vi "form FP title.vi"(2 "object ref":refnum<vi>) -> ()   [LabVIEW 2014, in "PTUtils.lvlib"]
doc: "Format the FrontPanel title by adding path do a settings file (if neccesary) and domain (or local CS system, if neccesary)"
uses:
  PTUtils.lvlib
  CS_Core/CSObj/CSObj.lvlib
  CS_Core/CSSystem/CSSystemLib/CSSystemLib.lvlib
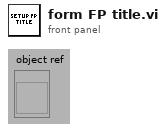
[diagram p1: front panel]
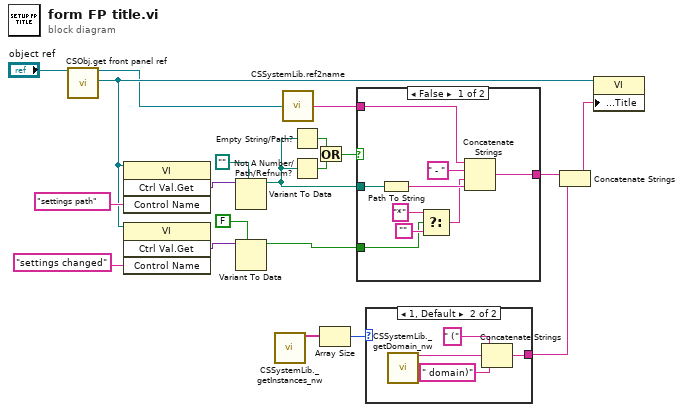
[diagram p0: block diagram]
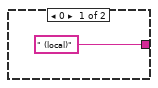
[diagram p3: hidden frame]
diagram:
  n1 = call "CSObj.get front panel ref.vi"("i ref in"="object ref") -> ("i ref out"=w1:refnum<vi>, "frontPanelRef"=w4:refnum<vi>)  [unwired: 16 in, 1 out]
  n2 = invoke class="VI" method="Ctrl Val.Get"(reference=w4, "Control Name"="settings path") -> ("Get Control Value Variant"=w9:variant)  [unwired: 2 in, 3 out]
  n3 = invoke class="VI" method="Ctrl Val.Get"(reference=w4, "Control Name"="settings changed") -> ("Get Control Value Variant"=w6:variant)  [unwired: 2 in, 3 out]
  n4 = Variant To Data(type=path "", Variant=w9) -> (data=w3:path)  [unwired: 1 in, 1 out]
  n5 = Variant To Data(type=FALSE, Variant=w6) -> (data=w2:bool)  [unwired: 1 in, 1 out]
  n6 = call "CSSystemLib._getInstances_nw.vi"() -> ("i list"=w14:string[])  [unwired: 18 in, 1 out]
  n7 = call "CSSystemLib.ref2name.vi"("obj refnum"=w1) -> ("name"=w19:string)
  n8 = Empty String/Path?(string/path=w3) -> (empty?=w12:bool)
  n9 = Not A Number/Path/Refnum?(number/path/refnum=w3) -> (NaN/Path/Refnum?=w11:bool)
  n10 = Or(x=w12, y=w11) -> (x .or. y?=w10:bool)
  n11 = Array Size(array=w14) -> (size(s)=w15:i32)
  n12 = case shown="False" w10 {
    tunnel: [w28 w30] -> w18
    tunnel: w19 -> [w27 w30]
    tunnel: w3 -> [w26 _]
    tunnel: w2 -> [w23 _]
    frame False {
      n13 = Path To String(path=w26) -> (string=w22:string)
      n14 = Select(t="*", s=w23, f="") -> (s? t:f=w21:string)
      n15 = Concatenate Strings(w27, " - ", w21, w22) -> (w28:string)
    }
    frame True {
    }
  }
  n16 = case shown="1, Default" w15 {
    tunnel: [" (local)" w32] -> w17
    frame 0 {
    }
    frame 1, Default {
      n17 = call "CSSystemLib._getDomain_nw.vi"() -> ("CSDomain"=w34:string)  [unwired: 18 in, 1 out]
      n18 = Concatenate Strings(" (", w34, " domain)") -> (w32:string)
    }
  }
  n19 = Concatenate Strings(w18, w17) -> (w16:string)
  n20 = property class="VI"(reference=w4, "Front Panel Window:Title"=w16) -> ()  [unwired: 1 in, 2 out]
